vi "Macanum Rotate.vi"(8 "Acceptable Error (in Degrees)":dbl=0.3, 9 "Rotation Speed":dbl=0.4, 10 "Heading Change (in Degrees)":dbl, 11 "RobotDriveDevRef":T2={"DevStatus"={"status"=FALSE, "code"=0, "source"=""}, "Motors[]"=[], "Square Inputs"=FALSE, "Max Output"=1.0, "Isochronous"=FALSE}) -> (0 "Actual Heading (in Degrees)":dbl(knob)=0.4937889940289276 scale=-180.0..180.0, 3 "RobotDriveDevRef":T2={"DevStatus"={"status"=FALSE, "code"=0, "source"=""}, "Motors[]"=[], "Square Inputs"=FALSE, "Max Output"=1.0, "Isochronous"=FALSE})   [LabVIEW 2011]
uses:
  <vilib>/Rock Robotics/WPI/RobotDrive/WPI_RobotDriveDevRef.ctl
  <vilib>/Rock Robotics/WPI/MotorControl/WPI_MotorControlDeviceRef.ctl
  <vilib>/Rock Robotics/SystemInterfaces/Typedef/FPGA_TypedefDigitalModule.ctl
  <vilib>/Rock Robotics/SystemInterfaces/DIO/FPGA_DIOPWMChannel.ctl
  <vilib>/Rock Robotics/WPI/PWM/WPI_PWMDeadband.ctl
  <vilib>/Rock Robotics/WPI/CAN/Jaguar/SubVIs/WPI_CANJaguar_ControlMode.ctl
  <vilib>/Rock Robotics/WPI/PWM/WPI_PWMTransform_ConPane.ctl
  Robot Global Data.vi
  <vilib>/addons/control/pid/pid.llb/PID (DBL).vi
  <vilib>/Rock Robotics/WPI/RobotDrive/WPI_RobotDriveMecanumDrive_Polar.vi
  <vilib>/addons/control/pid/NI_PID_pid.lvlib
panel:
  out "Rotation":dbl
  in  "StraightPID gains":T1={"proportional gain (Kc)"=0.025, "integral time (Ti, min)"=0.0, "derivative time (Td, min)"=0.0} {"derivative time (Td, min)" format="%.3f"; "integral time (Ti, min)" format="%.3f"; "proportional gain (Kc)" format="%.3f"}
  # "GYRO"
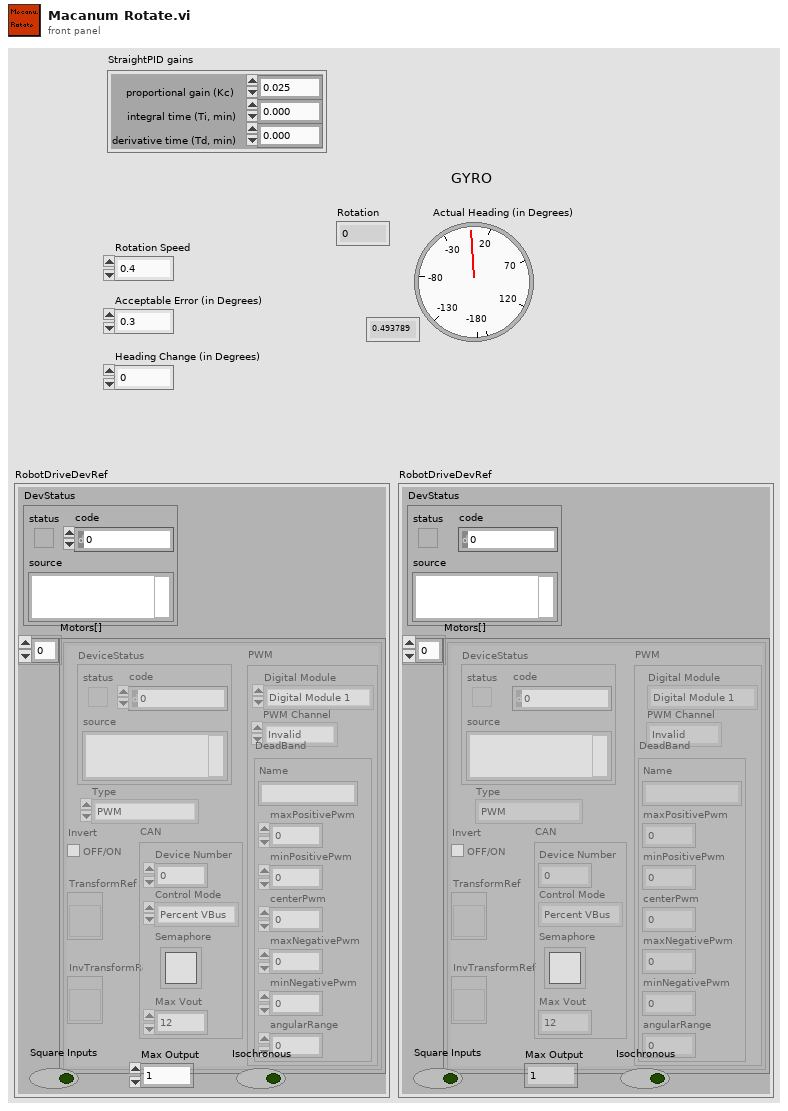
[diagram p1: front panel]
types:
  T1 = cluster{"proportional gain (Kc)":dbl, "integral time (Ti, min)":dbl, "derivative time (Td, min)":dbl}
  T2 = typedef "WPI_RobotDriveDevRef.ctl" = cluster{"DevStatus":errorcluster, "Motors[]":T3[], "Square Inputs":bool, "Max Output":dbl, "Isochronous":bool}
  T3 = typedef "WPI_MotorControlDeviceRef.ctl" = cluster{"DeviceStatus":errorcluster, "Type":enum16{"PWM", "CAN"}, "PWM":cluster{"Digital Module":T4, "PWM Channel":T5, "DeadBand":T6}, "CAN":cluster{"Device Number":u8, "Control Mode":T7, "Semaphore":T8, "Max Vout":dbl}, "Invert":bool, "TransformRef":T9, "InvTransformRef":T9}
  T4 = typedef "FPGA_TypedefDigitalModule.ctl" = enum16{"Digital Module 1", "Digital Module 2"}
  T5 = typedef "FPGA_DIOPWMChannel.ctl" = enum8{"PWM 1", "PWM 2", "PWM 3", "PWM 4", "PWM 5", "PWM 6", "PWM 7", "PWM 8", "PWM 9", "PWM 10", "Invalid"}
  T6 = typedef "WPI_PWMDeadband.ctl" = cluster{"Name":string, "maxPositivePwm":i32, "minPositivePwm":i32, "centerPwm":i32, "maxNegativePwm":i32, "minNegativePwm":i32, "angularRange":u16}
  T7 = typedef "WPI_CANJaguar_ControlMode.ctl" = enum8{"Percent VBus", "Current", "Speed", "Position", "Voltage"}
  T8 = typedef "Semaphore RefNum" = refnum<k1>
  T9 = typedef "WPI_PWMTransform_ConPane.ctl" = refnum<vi>
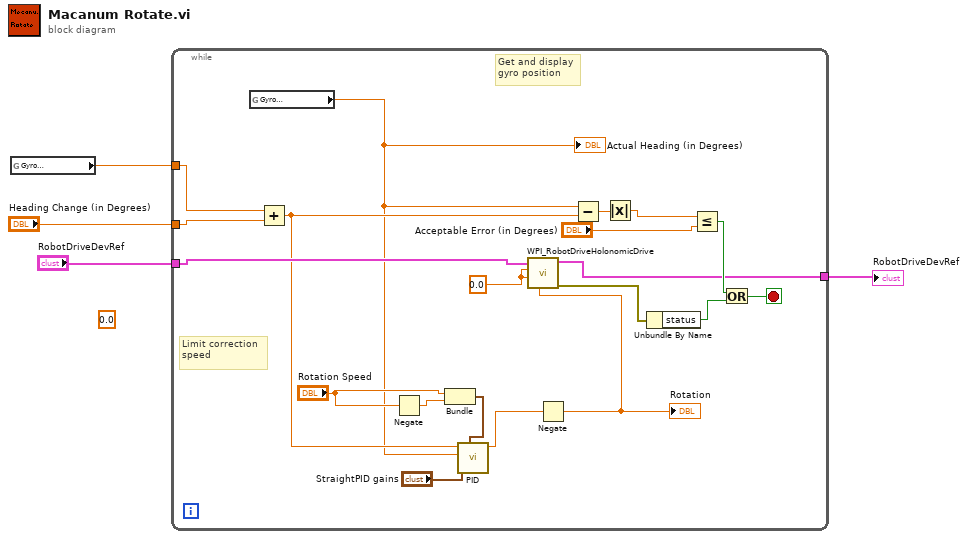
[diagram p0: block diagram]
diagram:
  (unwired) 0.0 ("Gyro\nAngle")
  n1 = global read "Robot Global Data.vi" "Gyro\nAngle"() -> (w1:dbl)
  n2 = while {
    tunnel: "RobotDriveDevRef" -> [w24]
    tunnel: "Heading Change (in Degrees)" -> [w7]
    tunnel: [w10] -> w2
    tunnel: w1 -> [w8]
    stop <- w23 stop-if-true
    w9 = 0.0 ("Magnitude")
    # "Limit correction\nspeed"
    # "Get and display\ngyro position"
    n3 = global read "Robot Global Data.vi" "Gyro\nAngle"() -> (w5:dbl)
    "Actual Heading (in Degrees)" <- w5
    n4 = Add(x=w8, y=w7) -> (x+y=w6:dbl)
    n5 = Negate(x="Rotation Speed") -> (-x=w18:dbl)
    n6 = Bundle("Rotation Speed"="Rotation Speed", w18) -> (w17:cluster{"Rotation Speed":dbl, dbl})  [unwired: 1 in]
    n7 = call-poly <vilib>:"PID.vi"("output range"=w17, "PID gains"="StraightPID gains", "process variable"=w5, "setpoint"=w6) -> ("output"=w21:dbl)  [unwired: 2 in, 5 out]
    n8 = Negate(x=w21) -> (-x=w11:dbl)
    "Rotation" <- w11
    n9 = call-poly <vilib>:"WPI_RobotDriveHolonomicDrive.vi"("Rotation"=w11, "Direction"=w9, "Magnitude"=w9, "RobotDriveDevRef"=w24) -> ("error out"=w22:errorcluster, "RobotDriveDevRef"=w10:T2)  [unwired: 2 in, 4 out]
    n10 = Subtract(x=w5, y=w6) -> (x-y=w16:dbl)
    n11 = Absolute Value(x=w16) -> (abs(x)=w15:dbl)
    n12 = Unbundle By Name(w22) -> ("status"=w13:bool)
    n13 = Less Or Equal?(x=w15, y="Acceptable Error (in Degrees)") -> (x <= y?=w12:bool)
    n14 = Or(x=w12, y=w13) -> (x .or. y?=w23:bool)
  }
  "RobotDriveDevRef" <- w2
